vi "Is Supported Cluster.vi"(11 "variant":variant) -> (2 "message type":string, 3 "supported?":bool)   [LabVIEW 2021, in "NI Measurement Plug-In SDK.lvlib"]
uses:
  NI Measurement Plug-In SDK.lvlib
  <vilib>/Utility/Data Type/NI_Data Type.lvlib
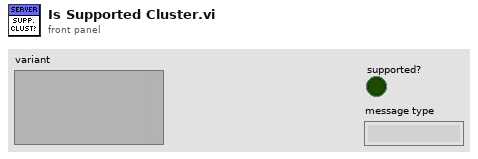
[diagram p1: front panel]
types:
  T1 = typedef "NI_Data Type.lvlib/Type Definition Info.ctl" = cluster{"Name":string, "Timestamp":u32}
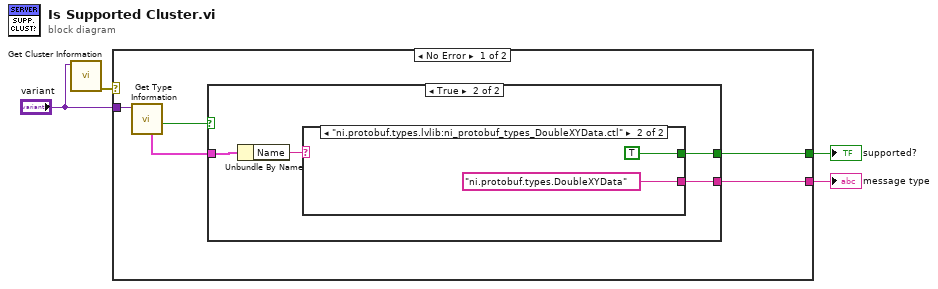
[diagram p0: block diagram]
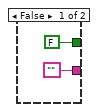
[diagram p2: hidden frame]
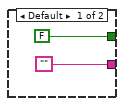
[diagram p3: hidden frame]
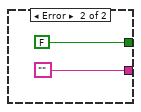
[diagram p4: hidden frame]
diagram:
  n1 = call <vilib>:"Get Cluster Information.vi"("variant"="variant") -> ("error out"=w3:errorcluster)  [unwired: 9 in, 1 out]
  n2 = case shown="No Error" w3 {
    tunnel: [w6 FALSE] -> w4
    tunnel: [w5 ""] -> w2
    tunnel: "variant" -> [w9 _]
    frame No Error {
      n3 = call <vilib>:"Get Type Information.vi"("variant"=w9) -> ("type definition"=w7:bool, "type definition info"=w8:T1)  [unwired: 6 in, 3 out]
      n4 = case shown="True" w7 {
        tunnel: w8 -> [_ w15]
        tunnel: [FALSE w13] -> w6
        tunnel: ["" w12] -> w5
        frame False {
        }
        frame True {
          n5 = Unbundle By Name(w15) -> ("Name"=w14:string)
          n6 = case shown="\"ni.protobuf.types.lvlib:ni_protobuf_types_DoubleXYData.ctl\"" w14 {
            tunnel: [FALSE TRUE] -> w13
            tunnel: ["" "ni.protobuf.types.DoubleXYData" ("message_type")] -> w12
            frame Default {
            }
            frame "ni.protobuf.types.lvlib:ni_protobuf_types_DoubleXYData.ctl" {
            }
          }
        }
      }
    }
    frame Error {
    }
  }
  "supported?" <- w4
  "message type" <- w2
